vi "BoneIP_Init.vi"(2 "error in":errorcluster, 3 "Task":enum16{"Init", "Close"}(ring)) -> (0 "error out":errorcluster)   [LabVIEW 2012]
uses:
  <userlib>/BotSpeak/VIs/Direct/BotSpeak_Control.ctl
panel:
  in  "Connection In":T1
  out "Connection Out":T1
  out "String":string
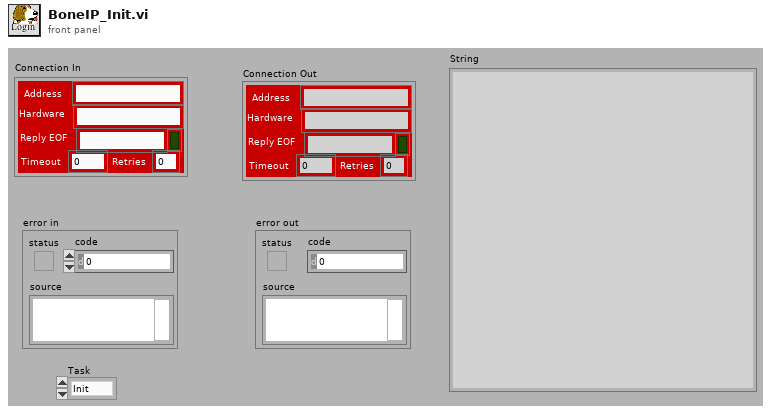
[diagram p1: front panel]
types:
  T1 = typedef "BotSpeak_Control.ctl" = cluster{"Address":string, "Reply EOF":string, "Hardware":string, "Retries":i8, "Timeout":i32, "Open?":bool}
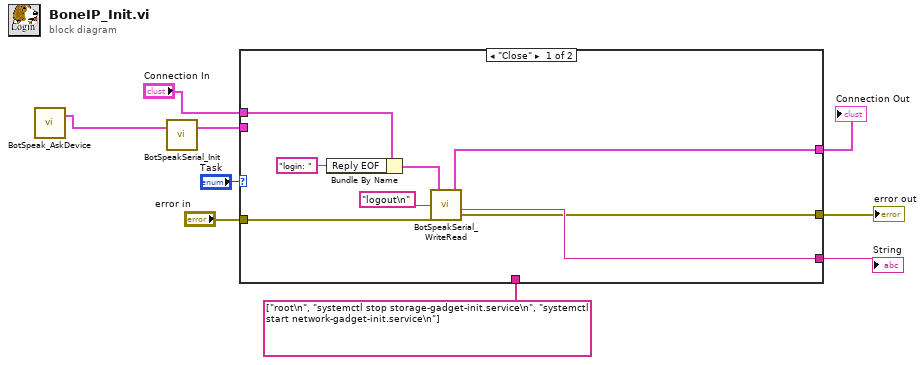
[diagram p0: block diagram]
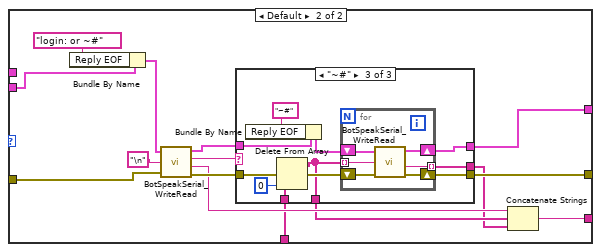
[diagram p2: hidden frame]
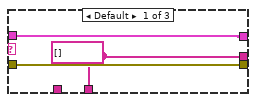
[diagram p3: hidden frame]
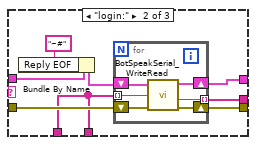
[diagram p4: hidden frame]
diagram:
  n1 = call <userlib>:"BotSpeak_AskDevice.vi"() -> ("Bot Settings out"=w1:T1)  [unwired: 3 in]
  n2 = call <userlib>:"BotSpeakSerial_Init.vi"("Bot Settings in"=w1) -> ("Bot Settings out"=w4:T1)  [unwired: 1 in, 1 out]
  n3 = case shown="\"Close\"" "Task" {
    tunnel: [w15 w32] -> w9
    tunnel: [w13 w30] -> w3
    tunnel: "Connection In" -> [w12 _]
    tunnel: [w16 w22] -> w8
    tunnel: "error in" -> [w14 w20]
    tunnel: string[] ["root\n", "systemctl stop storage-gadget-init.service\n", "systemctl start network-gadget-init.service\n"] -> [_ w19]
    tunnel: w4 -> [_ w18]
    frame "Close" {
      n4 = Bundle By Name(cluster=w12, "Reply EOF"="login: " ("Bot Settings.Reply EOF")) -> (w11:T1)
      n5 = call <userlib>:"BotSpeakSerial_WriteRead.vi"("error In"=w14, "To Write"="logout\n" ("String To Send"), "Bot Settings in"=w11) -> ("error out"=w15:errorcluster, "Reply"=w16:string, "Bot Settings out"=w13:T1)  [unwired: 1 out]
    }
    frame Default {
      n6 = Bundle By Name(cluster=w18, "Reply EOF"="login: or ~#" ("Status String")) -> (w27:T1)
      n7 = call <userlib>:"BotSpeakSerial_WriteRead.vi"("error In"=w20, "To Write"="\n" ("Status String"), "Bot Settings in"=w27) -> ("error out"=w31:errorcluster, "Reply"=w25:string, "Reply EOF"=w21:string, "Bot Settings out"=w29:T1)
      n8 = case shown="\"~#\"" w21 {
        tunnel: [w34 w43 w59] -> w32
        tunnel: w31 -> [w34 w42 w58]
        tunnel: [w35 w41 w57] -> w30
        tunnel: w29 -> [w35 w38 w54]
        tunnel: [w33 w36 w51] -> w24
        tunnel: [w33 w37 w53] -> w23
        tunnel: w19 -> [_ w36 w52]
        frame Default {
          w33 = string[] []
        }
        frame "login:" {
          n9 = Bundle By Name(cluster=w38, "Reply EOF"="~#" ("Status String")) -> (w40:T1)
          n10 = for {
            tunnel: w36 -> [w45] mode=indexing
            tunnel: [w44] -> w37 mode=indexing
            shift-right: [w47] -> w41
            shift-left: w40 -> [w46]
            shift-right: [w49] -> w43
            shift-left: w42 -> [w48]
            n11 = call <userlib>:"BotSpeakSerial_WriteRead.vi"("error In"=w48, "To Write"=w45, "Bot Settings in"=w46) -> ("error out"=w49:errorcluster, "Reply"=w44:string, "Bot Settings out"=w47:T1)  [unwired: 1 out]
          }
        }
        frame "~#" {
          n12 = Bundle By Name(cluster=w54, "Reply EOF"="~#" ("Status String")) -> (w56:T1)
          n13 = Delete From Array(array=w52, index=0) -> (array with subset deleted=w51:string[])  [unwired: 1 in, 1 out]
          n14 = for {
            tunnel: [w61] -> w53 mode=indexing
            shift-right: [w63] -> w57
            shift-left: w56 -> [w62]
            shift-right: [w65] -> w59
            shift-left: w58 -> [w64]
            tunnel: w51 -> [w60] mode=indexing
            n15 = call <userlib>:"BotSpeakSerial_WriteRead.vi"("error In"=w64, "To Write"=w60, "Bot Settings in"=w62) -> ("error out"=w65:errorcluster, "Reply"=w61:string, "Bot Settings out"=w63:T1)  [unwired: 1 out]
          }
        }
      }
      n16 = Concatenate Strings(w25, w24, w23) -> (w22:string)
    }
  }
  "error out" <- w9
  "String" <- w8
  "Connection Out" <- w3
